vi "FRCts20_Backend_Request_PUT.vi"(6 "Message Attributes":T4, 8 "error in (no error)":errorcluster, 10 "Data":string, 11 "Engine_Refnums":T1) -> (0 "error out":errorcluster)   [LabVIEW 2013, in "FRCts20_Backend_Engine.lvlib"]
doc: "Sets the status of a request to closed, in work, or open. Called by the Request API. Expects a request index and status."
uses:
  FRCts20_Backend_Engine.lvlib
  Dependencies/Keyed Array/KeyedArray.ctl
  FRCts20_Backend_EngineRefnums.ctl
  INI_Accessor/FRCts20_Backend_INI Controller.lvclass
  Dependencies/AMC/_SubVIs/TypeDefs/Message Queue.ctl
  Dependencies/AMC/_SubVIs/TypeDefs/Message.ctl
  <vilib>/addons/database/Connection.llb/Conn ObjectReference.ctl
  FRCts20_Backend_API/FRCts20_Backend_API_Request.ctl
  FRCts20_Backend_API/FRCts20_Backend_API_Status.ctl
  FRCts20_Backend_FGVOperation.ctl
  FRCts20_Backend_API/FRCts20_Backend_API.lvlib
  Dependencies/Keyed Array/Tools_KeyedArray.lvlib
  Dependencies/AMC/AMC.lvlib
  <vilib>/addons/database/NI_Database_API.lvlib
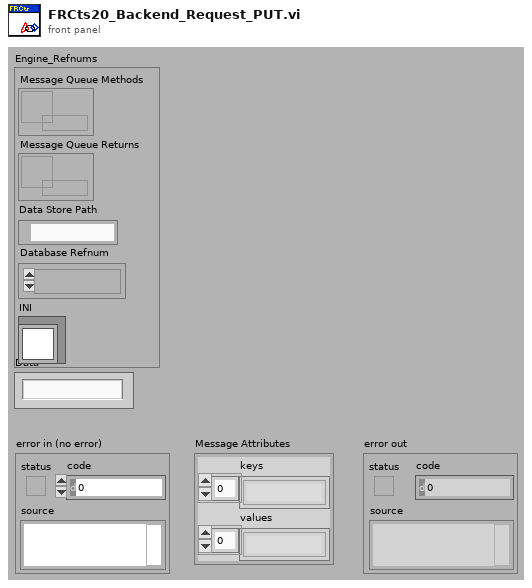
[diagram p1: front panel]
types:
  T1 = typedef "FRCts20_Backend_Engine.lvlib/FRCts20_Backend_EngineRefnums.ctl" = cluster{"Message Queue Methods":T2, "Message Queue Returns":T2, "Data Store Path":path, "Database Refnum":T3, "INI":refnum<class "FRCts20_Backend_INI Controller.lvclass">}
  T2 = typedef "AMC.lvlib/Message Queue.ctl" = refnum<queue>
  T3 = typedef "NI_Database_API.lvlib/Conn ObjectReference.ctl" = refnum<k1>
  T4 = typedef "Tools_KeyedArray.lvlib/KeyedArray.ctl" = cluster{"keys":string[], "values":string[]}
  T5 = typedef "FRCts20_Backend_Engine.lvlib/FRCts20_Backend_FGVOperation.ctl" = enum16{"Initialize", "EnqueueMessage", "EnqueueDataReturn", "FlushMessage", "FlushDataReturn"}
  T6 = typedef "FRCts20_Backend_API.lvlib/FRCts20_Backend_API_Request.ctl" = cluster{"Request Index":u32, "Description":string, "Status":T7, "Open Date":timestamp, "Last Update":timestamp, "Closed Date":timestamp, "Notes":cluster{"Note Index":u32, "Text":string, "Time Entered":timestamp, "Author":string, "Solution":bool}[], "Team Index":u32, "APIReturn":string}
  T7 = typedef "FRCts20_Backend_API.lvlib/FRCts20_Backend_API_Status.ctl" = enum16{"Open", "In Work", "Closed"}
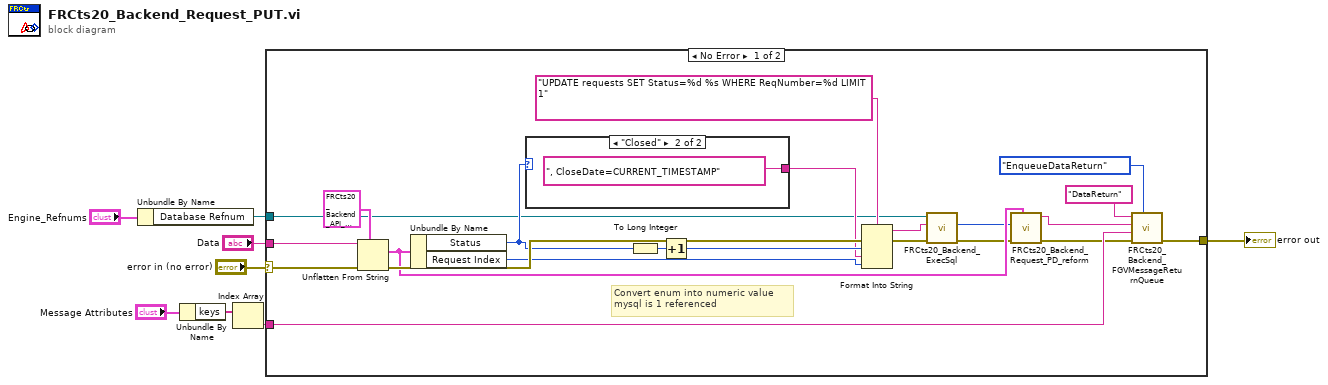
[diagram p0: block diagram]
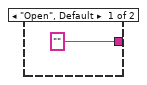
[diagram p2: hidden frame]
diagram:
  n1 = Unbundle By Name("Engine_Refnums") -> ("Database Refnum"=w5:T3)
  n2 = Unbundle By Name("Message Attributes") -> ("keys"=w2:string[])
  n3 = Index Array(array=w2) -> (element=w1:string)  [unwired: 1 in]
  n4 = case shown="No Error" "error in (no error)" {
    selector: "error in (no error)" -> [w27 w33]
    tunnel: [w30 w33] -> w7
    tunnel: w5 -> [w13 _]
    tunnel: "Data" -> [w28 _]
    tunnel: w1 -> [w29 _]
    frame No Error {
      # "Convert enum into numeric value\nmysql is 1 referenced"
      n5 = Unflatten From String(type=T6 {"Request Index"=0, "Description"="", "Status"=enum."Open", "Open Date"=timestamp(0 s since 1904-01-01), "Last Update"=timestamp(0 s since 1904-01-01), "Closed Date"=timestamp(0 s since 1904-01-01), "Notes"=[], "Team Index"=0, "APIReturn"=""} ("Request"), binary string=w28, error in (no error)=w27) -> (value=w14:T6, error out=w26:errorcluster)  [unwired: 2 in, 1 out]
      n6 = Unbundle By Name(w14) -> ("Status"=w20:T7, "Request Index"=w22:u32)
      n7 = case shown="\"Closed\"" w20 {
        tunnel: ["" ", CloseDate=CURRENT_TIMESTAMP"] -> w21
        frame "Open", Default {
        }
        frame "Closed" {
        }
      }
      n8 = To Long Integer(number=w20) -> (32bit integer=w19:i32)
      n9 = Increment(x=w19) -> (x+1=w24:i32)
      n10 = Format Into String(format string="UPDATE requests SET Status=%d %s WHERE ReqNumber=%d LIMIT 1", error in=w26, w24, w21, w22) -> (resulting string=w12:string, error out=w11:errorcluster)  [unwired: 1 in]
      n11 = call "FRCts20_Backend_ExecSql.vi"("error in (no error)"=w11, "format string"=w12, "Refnum in"=w13) -> ("error out"=w9:errorcluster, "rows affected"=w10:i32)  [unwired: 6 in, 1 out]
      n12 = call "FRCts20_Backend_Request_PD_reform.vi"("Request"=w14, "error in (no error)"=w9, "rows affected"=w10) -> ("error out"=w15:errorcluster, "data string"=w16:string)  [unwired: 7 in]
      n13 = call "FRCts20_Backend_FGVMessageReturnQueue.vi"("Operation"=FRCts20_Backend_FGVOperation."EnqueueDataReturn", "error in (no error)"=w15, "Key"=w29, "Message Value"=w16, "Message Name"="DataReturn") -> ("error out"=w30:errorcluster)  [unwired: 5 in, 1 out]
    }
    frame Error {
    }
  }
  "error out" <- w7
